vi "FGV Modbus Kommunikation OO.vi"(5 "Aktionen":T1=enum."lesen", 6 "error in":errorcluster caption="error out", 8 "IP-Adresse":string, 9 "Steuerung PNS (Eingang)":refnum<class "Steuerung PNS.lvclass">) -> (0 "Fehler (Ausgang)":errorcluster, 1 "Index":u8, 2 "Case Nr.":u8, 3 "Steuerung PNS (Ausgang)":refnum<class "Steuerung PNS.lvclass">, 4 "maxLoop":u8=10)   [LabVIEW 2020, in "PNS.lvlib" / "Komm Modbus.lvlib"]
uses:
  Komm Modbus.lvlib
  Aktionen FGV Komm MB.ctl
  ObjektKlassen/Steuerung PNS/Steuerung PNS.lvclass
  Aktionen FGV Grenzwerte.ctl
  Aktionen FGV Istwerte.ctl
  Aktion FGV AO PNS.ctl
  Aktion FGV Ventile manuell steuern.ctl
  Aktionen FGV Loopkennung.ctl
  PNS.lvlib
  Allgemein/allgemeine Sub-VIs.lvlib
  Modbus TypDef.lvlib
panel:
  out "x-y":u32
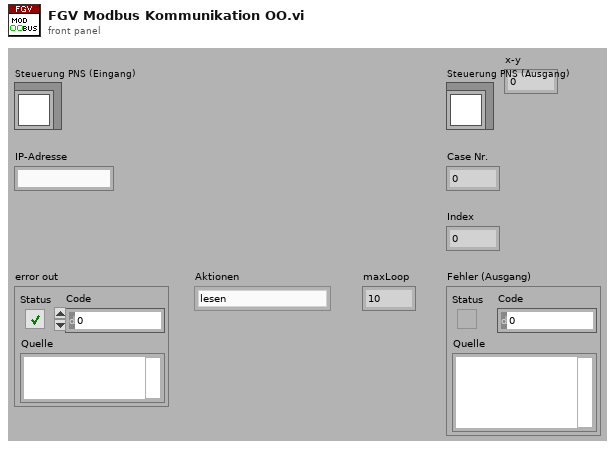
[diagram p1: front panel]
types:
  T1 = typedef "PNS.lvlib/Komm Modbus.lvlib/Modbus TypDef.lvlib/Aktionen FGV Komm MB.ctl" = enum16{"initialisieren", "lesen", "Verbindung herstellen", "Verbindung beenden", "Komm Modbus", "Sollwerte vorgeben", "change lang"}
  T2 = typedef "PNS.lvlib/Aktion FGV Ventile manuell steuern.ctl" = enum16{"lesen", "Ventile schalten"}
  T3 = typedef "PNS.lvlib/Aktion FGV AO PNS.ctl" = enum16{"lesen", "schreiben"}
  T4 = typedef "PNS.lvlib/Aktionen FGV Istwerte.ctl" = enum16{"lesen", "initialisieren", "schreiben", "Störungen"}
  T5 = typedef "PNS.lvlib/Aktionen FGV Grenzwerte.ctl" = enum16{"lesen", "Grenzw. schreiben", "Anweisungscode", "IP-Adresse", "laden", "speichern", "Anweisungscode vorgeben"}
  T6 = typedef "PNS.lvlib/Aktionen FGV Loopkennung.ctl" = enum16{"lesen", "schreiben"}
  T7 = typedef "Steuerung PNS.lvclass/Alarme.ctl" = cluster{"Alarm Filter max":u16, "Alarm Filter min":u16, "Alarm Ventilplatte max":u16, "Alarm Ventilplatte min":u16, "Alarm HL1 max":u16, "Alarm HL1 min":u16, "Alarm HL2 max":u16, "Alarm HL2 min":u16, "Alarm HL3 max":u16, "Alarm HL3 min":u16, "Alarm HL4 max":u16, "Alarm HL4 min":u16, "Alarm HL5 max":u16, "Alarm HL5 min":u16, "Alarm HL6 max":u16, "Alarm HL6 min":u16}
  T8 = typedef "Steuerung PNS.lvclass/Regler.ctl" = cluster{"Istwert":i16, "Sollwert":i16, "Alarm MIN":i16, "Alarm MAX":i16, "Regler sperren":i16, "Analog Ausgang":i16}[]
  T9 = typedef "Steuerung PNS.lvclass/Anlegengrenzwerte PNS.ctl" = cluster{"Filter:":T10, "Ventilplatte:":T10, "Heizleitung 1:":T10, "Heizleitung 2:":T10, "Heizleitung 3:":T10, "Heizleitung 4:":T10, "Heizleitung 5:":T10, "Heizleitung 6:":T10}
  T10 = typedef "Steuerung PNS.lvclass/Anlagengrenzwerte Parameteranzeige.ctl" = cluster{"Sollwert":T11, "Warn-Min":T11, "Warn-Max":T11, "Abschalt-Min":T11, "Abschalt-Max":T11, "Regler":u16, "AnlagenParameter":string}
  T11 = typedef "Zahlen-Eingabefeld.ctl" = sgl
  T12 = typedef "PNS.lvlib/PNS Geraetekennung.ctl" = cluster{"Loops":string[], "Gerätetype":string, "Loopkennung":u16[], "Seriennummer":string, "Geraetekennung":u16, "SoftWare Version":string, "LP Kennung":u16}
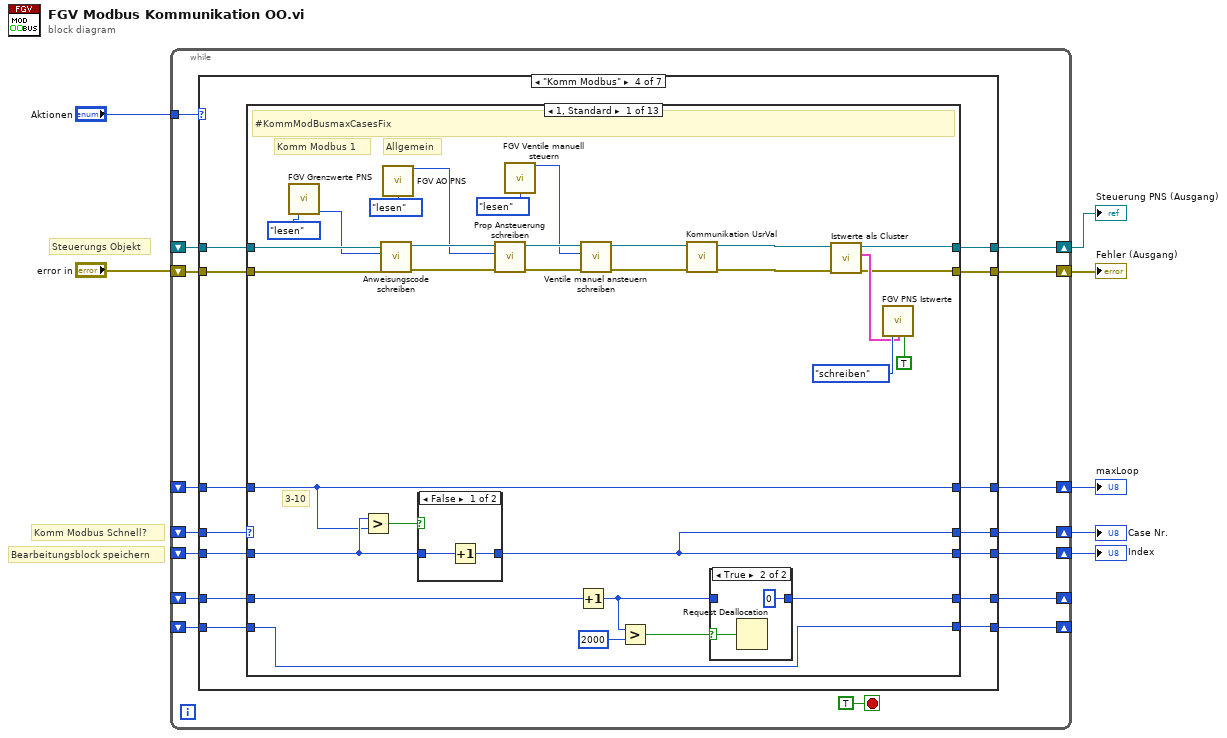
[diagram p0: block diagram]
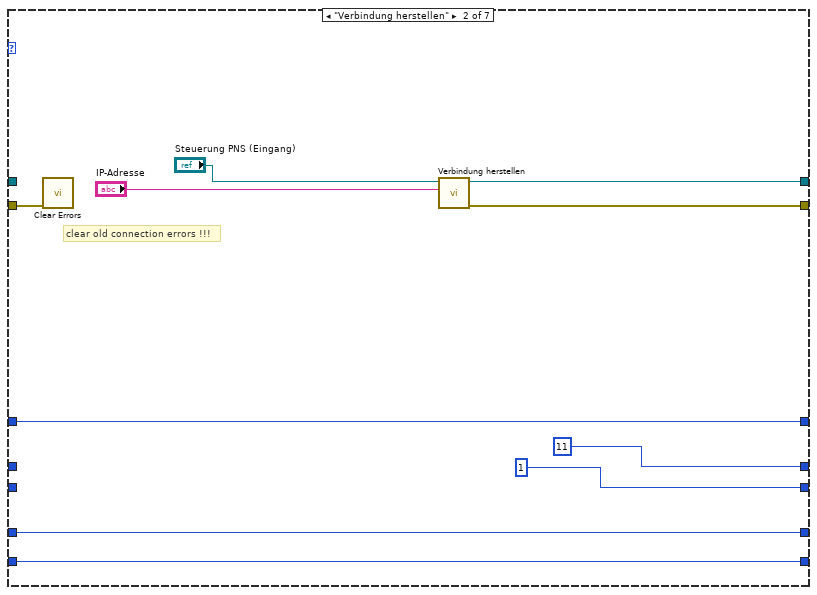
[diagram p3: hidden frame]
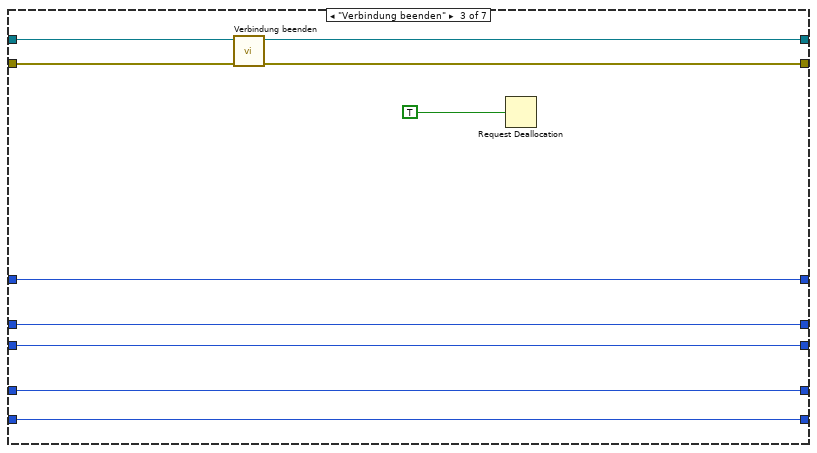
[diagram p4: hidden frame]
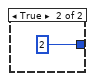
[diagram p6: hidden frame]
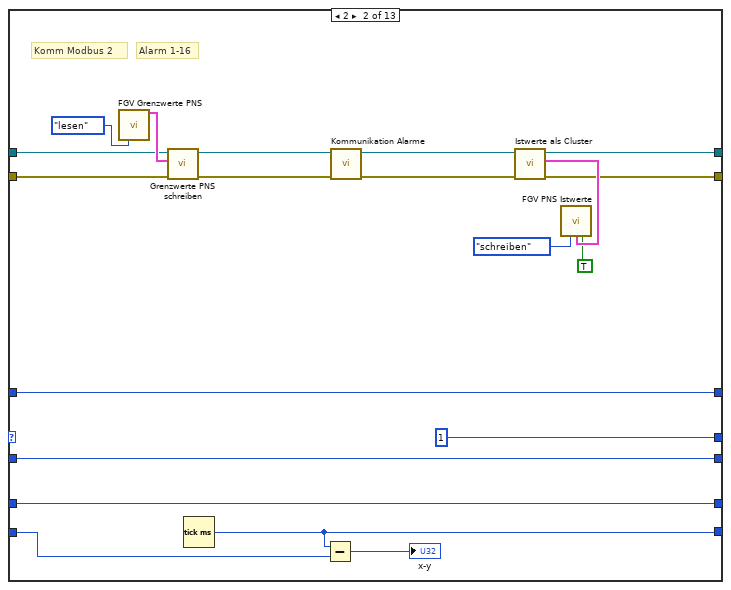
[diagram p7: hidden frame]
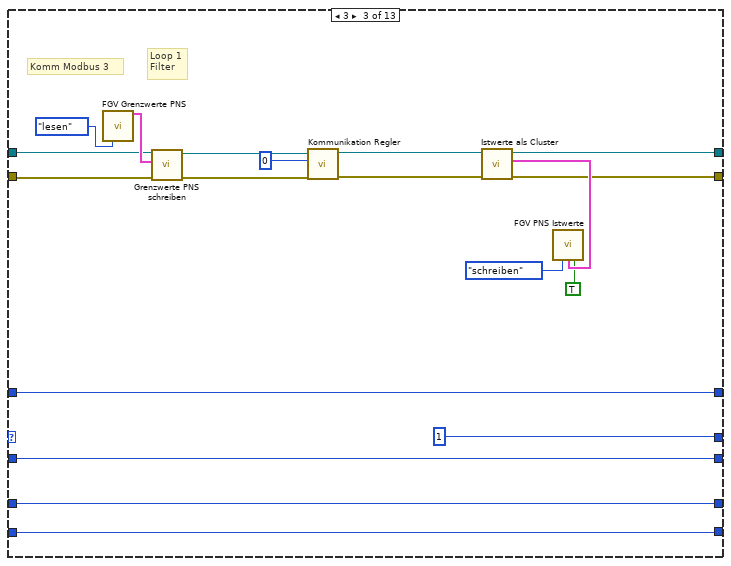
[diagram p8: hidden frame]
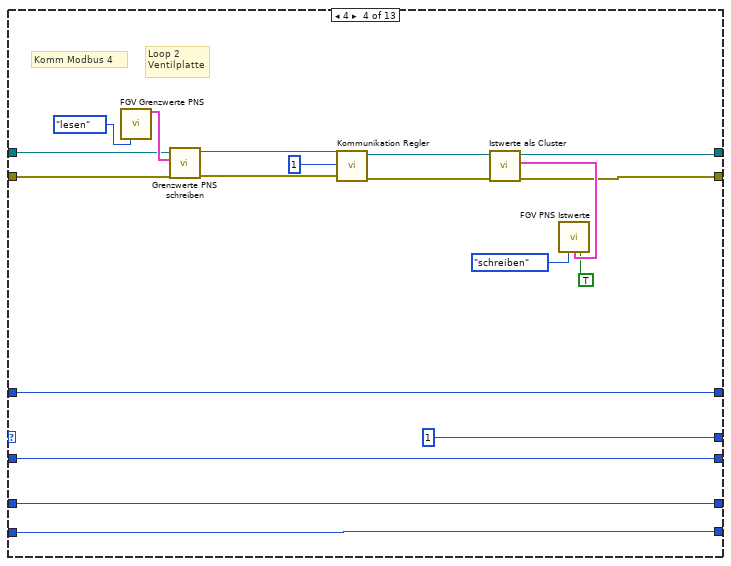
[diagram p9: hidden frame]
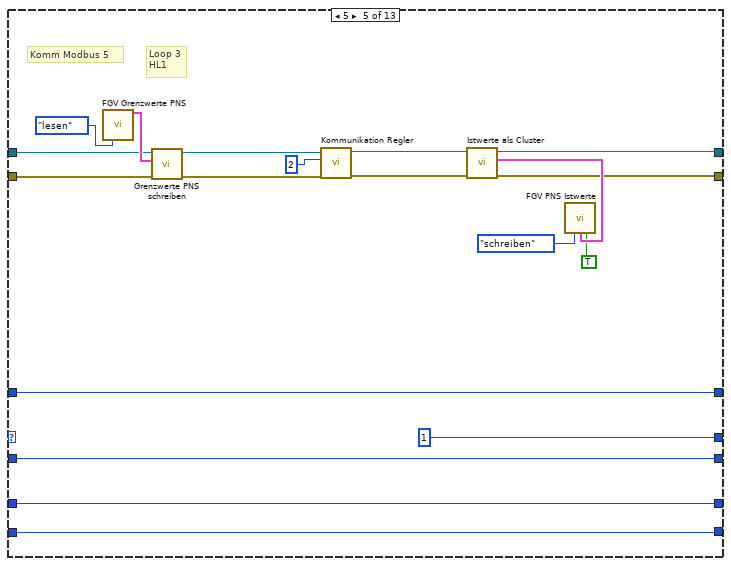
[diagram p10: hidden frame]
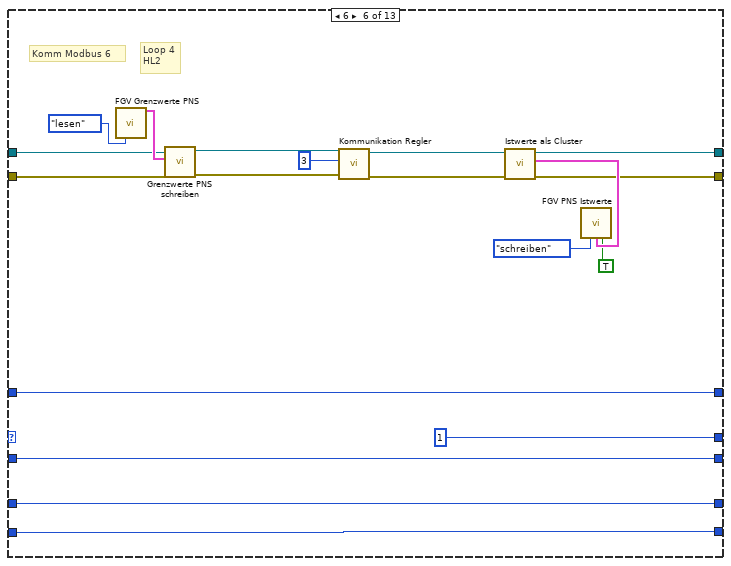
[diagram p11: hidden frame]
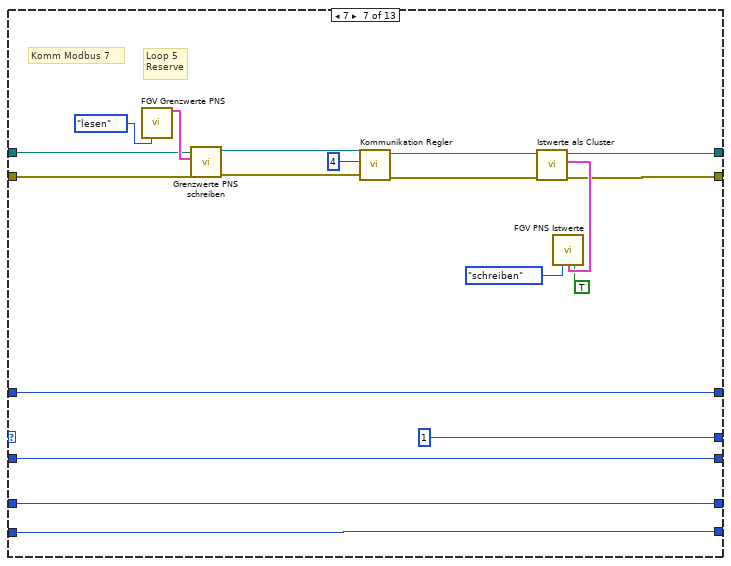
[diagram p12: hidden frame]
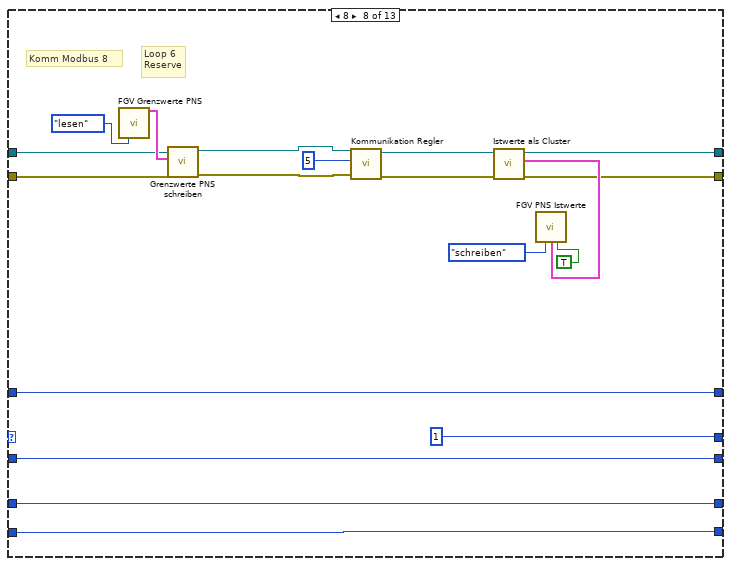
[diagram p13: hidden frame]
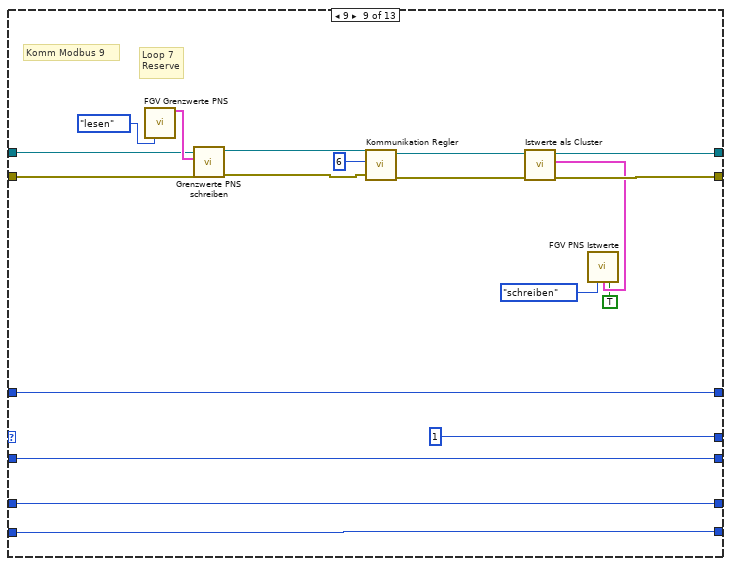
[diagram p14: hidden frame]
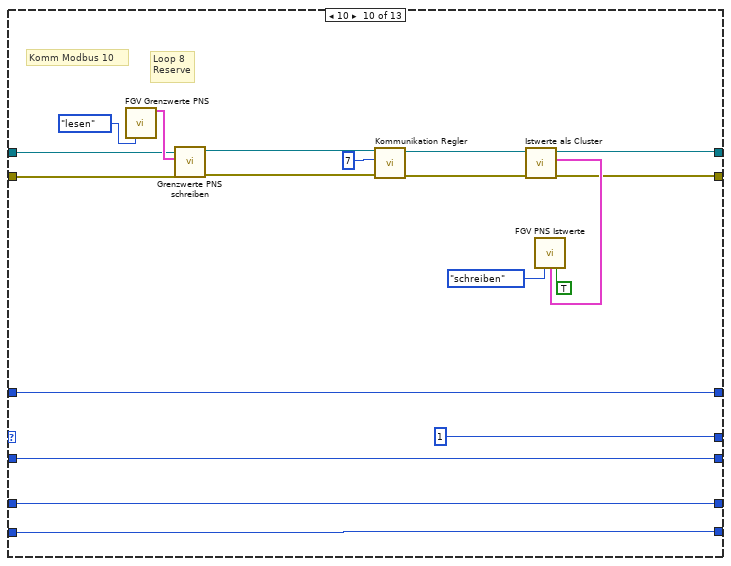
[diagram p15: hidden frame]
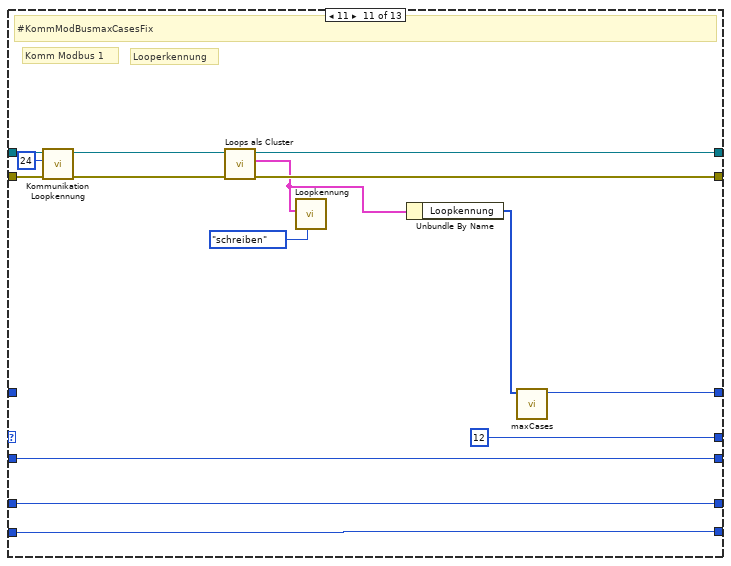
[diagram p16: hidden frame]
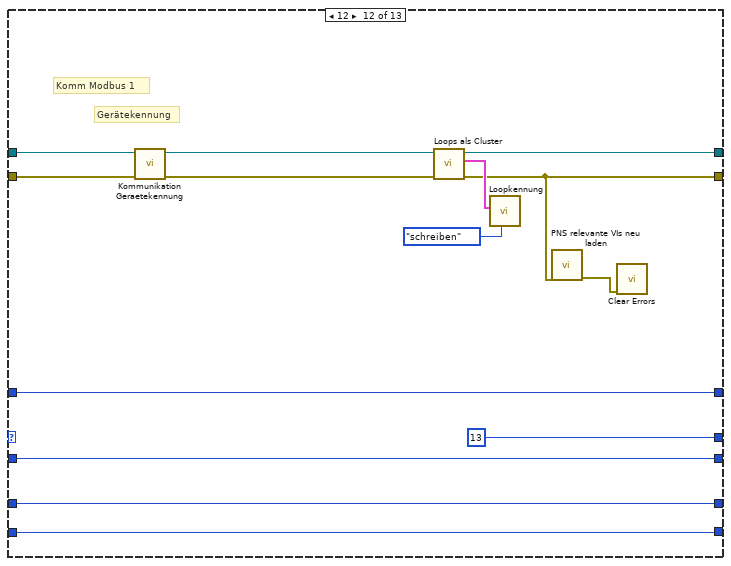
[diagram p17: hidden frame]
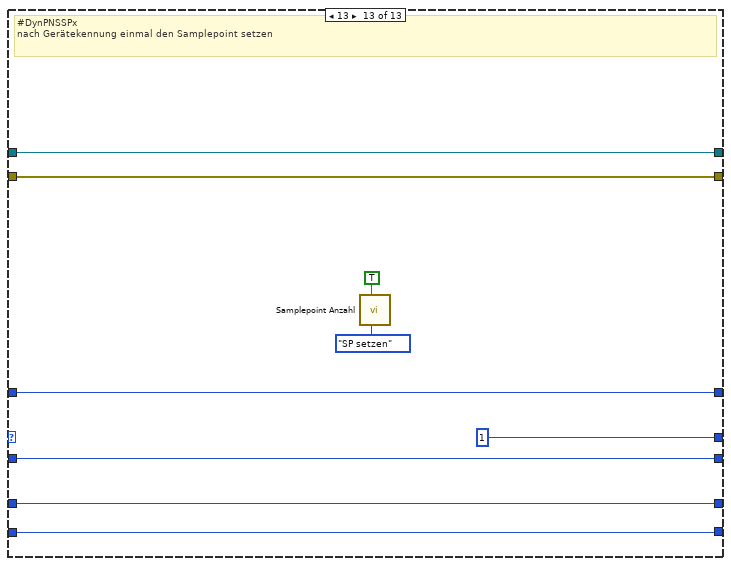
[diagram p18: hidden frame]
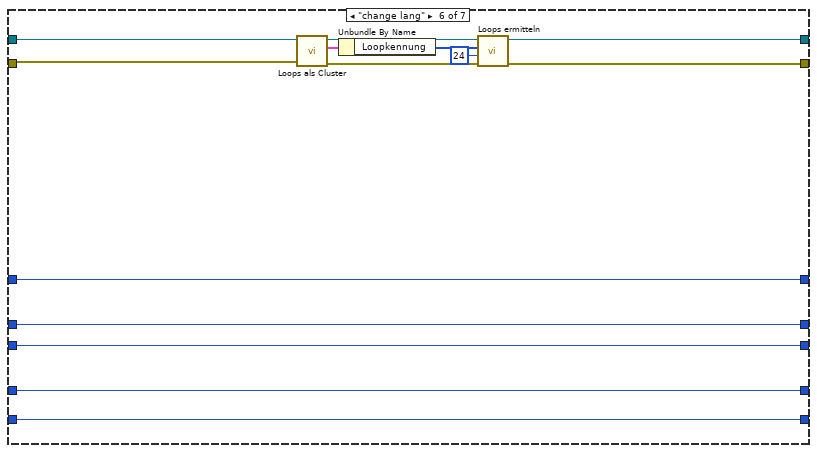
[diagram p20: hidden frame]
diagram:
  # "Bearbeitungsblock speichern"
  # "Komm Modbus Schnell?"
  # "Steuerungs Objekt"
  n1 = while {
    tunnel: "Aktionen" -> [w22]
    shift-right: [w21] -> w3
    shift-left: _ -> [w19]
    shift-right: [w20] -> w6
    shift-left: "error in" -> [w18]
    shift-right: [w16] -> w5
    shift-left: _ -> [w17]
    shift-right: [w15] -> w4
    shift-left: _ -> [w14]
    shift-right: [w13] -> _
    shift-left: _ -> [w12]
    shift-right: [w11] -> _
    shift-left: _ -> [w10]
    shift-right: [w9] -> w2
    shift-left: _ -> [w8]
    stop <- TRUE stop-if-true
    n2 = case shown="\"Komm Modbus\"" w22 {
      tunnel: [w30 w35 w45 w53 w318 w323 w338] -> w21
      tunnel: [w29 w36 w43 w64 w317 w321 w337] -> w20
      tunnel: w19 -> [w30 _ w42 w63 w318 w324 w338]
      tunnel: w18 -> [w29 w32 w44 w54 w317 w322 w337]
      tunnel: w17 -> [w28 _ w50 w59 w316 w331 w336]
      tunnel: [w28 u8 11 ("x") w50 w61 w316 w331 w336] -> w16
      tunnel: w14 -> [w27 _ w49 w62 w315 w330 w335]
      tunnel: [w27 u8 1 ("x") w49 w60 w315 w330 w335] -> w15
      tunnel: [w26 w39 w47 w57 w314 w332 w339] -> w13
      tunnel: w12 -> [w26 w39 w47 w58 w314 w332 w339]
      tunnel: [w25 w37 w46 w56 w313 w329 w334] -> w11
      tunnel: w10 -> [w25 w37 w46 w55 w313 w329 w334]
      tunnel: [w24 w31 w41 w52 w312 w319 w333] -> w9
      tunnel: w8 -> [w24 w31 w41 w51 w312 w319 w333]
      frame "lesen", Default {
      }
      frame "Verbindung herstellen" {
        # "clear old connection errors !!!"
        n3 = call <vilib>:"Clear Errors.vi"("error in (no error)"=w32) -> ()  [unwired: 5 in, 2 out]
        n4 = call "Verbindung herstellen.vi"("IP Adresse"="IP-Adresse", "Steuerung PNS (Eingang)"="Steuerung PNS (Eingang)") -> ("error out"=w36:errorcluster, "Steuerung PNS (Ausgang)"=w35:refnum<class "Steuerung PNS.lvclass">)  [unwired: 8 in]
      }
      frame "Verbindung beenden" {
        n5 = call "Verbindung beenden.vi"("error in (no error)"=w44, "Steuerung PNS Eingang"=w42) -> ("error out"=w43:errorcluster, "Steuerung PNS Ausgang"=w45:refnum<class "Steuerung PNS.lvclass">)  [unwired: 8 in]
        n6 = Request Deallocation(TRUE ("Flag")) -> ()
      }
      frame "Komm Modbus" {
        n7 = case shown="1, Standard" w59 {
          tunnel: [w78 w104 w124 w143 w162 w181 w200 w219 w240 w257 w278 w291 w306] -> w64
          tunnel: w63 -> [w85 w112 w132 w151 w170 w189 w208 w227 w246 w265 w284 w298 w307]
          tunnel: w62 -> [w93 w119 w138 w157 w176 w195 w214 w233 w252 w271 w287 w301 w310]
          tunnel: [w95 u8 1 ("x") u8 1 ("x") u8 1 ("x") u8 1 ("x") u8 1 ("x") u8 1 ("x") u8 1 ("x") u8 1 ("x") u8 1 ("x") u8 12 ("x") u8 13 ("x") u8 1 ("x")] -> w61
          tunnel: [w95 w119 w138 w157 w176 w195 w214 w233 w252 w271 w287 w301 w310] -> w60
          tunnel: w58 -> [w92 w120 w140 w159 w178 w197 w216 w235 w254 w273 w288 w302 w311]
          tunnel: [w89 w120 w140 w159 w178 w197 w216 w235 w254 w273 w288 w302 w311] -> w57
          tunnel: [w87 w118 w137 w156 w175 w194 w213 w232 w251 w270 w285 w299 w308] -> w56
          tunnel: w55 -> [w87 w116 w137 w156 w175 w194 w213 w232 w251 w270 w285 w299 w308]
          tunnel: w54 -> [w84 w109 w129 w149 w169 w188 w207 w226 w245 w264 w283 w297 w306]
          tunnel: [w82 w108 w128 w147 w166 w185 w204 w223 w242 w261 w280 w295 w307] -> w53
          tunnel: [w75 w102 w122 w141 w160 w179 w198 w217 w236 w255 w274 w289 w303] -> w52
          tunnel: w51 -> [w75 w102 w122 w141 w160 w179 w198 w217 w236 w255 _ w289 w303]
          frame 1, Default {
            # "3-10"
            # "Allgemein"
            # "Komm Modbus 1"
            # "#KommModBusmaxCasesFix"
            n8 = call "FGV Grenzwerte PNS.vi"("Aktionen FGV Grenzwerte"=Aktionen_FGV_Grenzwerte."lesen") -> ("Anweisungscode"=w76:u16)  [unwired: 12 in, 2 out]
            n9 = Greater?(x=w93, y=w75) -> (0:w94:bool)
            n10 = call-dynamic "Anweisungscode schreiben.vi"("error in (no error)"=w84, "Anweisungscode"=w76, "Steuerung PNS (Eingang)"=w85) -> ("error out"=w73:errorcluster, "Steuerung PNS (Ausgang)"=w74:refnum<class "Steuerung PNS.lvclass">)  [unwired: 7 in]
            n11 = call "FGV AO PNS.vi"("Aktion"=Aktion_FGV_AO_PNS."lesen") -> ("AO PROP"=w71:u16)  [unwired: 13 in, 1 out]
            n12 = case shown="False" w94 {
              tunnel: w93 -> [w100 _]
              tunnel: [w99 u8 2 ("Index")] -> w95
              frame False {
                n13 = Increment(x=w100) -> (x+1=w99:u8)
              }
              frame True {
              }
            }
            n14 = call-dynamic "Prop Ansteuerung schreiben.vi"("error in (no error)"=w73, "Propansteuerung"=w71, "Steuerung PNS (Eingang)"=w74) -> ("error out"=w68:errorcluster, "Steuerung PNS (Ausgang)"=w70:refnum<class "Steuerung PNS.lvclass">)  [unwired: 7 in]
            n15 = call "FGV Ventile manuell steuern.vi"("Aktion"=Aktion_FGV_Ventile_manuell_steuern."lesen") -> ("Ventile schalten"=w65:u32)  [unwired: 13 in, 1 out]
            n16 = Increment(x=w92) -> (x+1=w90:i32)
            n17 = call-dynamic "Ventile manuel ansteuern schreiben.vi"("error in (no error)"=w68, "Ventile steuern"=w65, "Steuerung PNS (Eingang)"=w70) -> ("error out"=w67:errorcluster, "Steuerung PNS (Ausgang)"=w69:refnum<class "Steuerung PNS.lvclass">)  [unwired: 7 in]
            n18 = Greater?(x=w90, y=2000) -> (0:w88:bool)
            n19 = call "Kommunikation UsrVal.vi"("error in (no error)"=w67, "Steuerung PNS Eingang"=w69) -> ("error out"=w79:errorcluster, "Steuerung PNS Ausgang"=w86:refnum<class "Steuerung PNS.lvclass">)  [unwired: 7 in, 1 out]
            n20 = case shown="True" w88 {
              selector: w88 -> [_ w97]
              tunnel: w90 -> [w96 _]
              tunnel: [w96 0] -> w89
              frame False {
              }
              frame True {
                n21 = Request Deallocation(w97) -> ()
              }
            }
            n22 = call "Istwerte als Cluster.vi"("error in (no error)"=w79, "Steuerung PNS Eingang"=w86) -> ("error out"=w78:errorcluster, "Cluster"=w80:cluster{"UsrVal":u16[], "Alarm":T7, "Regler":T8}, "Steuerung PNS Ausgang"=w82:refnum<class "Steuerung PNS.lvclass">)  [unwired: 7 in]
            n23 = call "FGV PNS Istwerte.vi"("Aktionen"=Aktionen_FGV_Istwerte."schreiben", "Cluster"=w80, "Speicher Freigabe"=TRUE) -> ()  [unwired: 9 in, 4 out]
          }
          frame 2 {
            # "Alarm 1-16"
            # "Komm Modbus 2"
            n24 = call "FGV Grenzwerte PNS.vi"("Aktionen FGV Grenzwerte"=Aktionen_FGV_Grenzwerte."lesen") -> ("Grenzwerte PNS 2"=w114:T9)  [unwired: 12 in, 2 out]
            n25 = call-dynamic "Grenzwerte PNS schreiben.vi"("error in (no error)"=w109, "Grenzwerte PNS"=w114, "Steuerung PNS (Eingang)"=w112) -> ("error out"=w110:errorcluster, "Steuerung PNS (Ausgang)"=w111:refnum<class "Steuerung PNS.lvclass">)  [unwired: 7 in]
            n26 = Tick Count (ms)() -> (millisecond timer value=w118:u32)
            n27 = Subtract(x=w118, y=w116) -> (x-y=→"x-y":u32)
            n28 = call "Kommunikation Alarme.vi"("error in (no error)"=w110, "Steuerung PNS Eingang"=w111) -> ("error out"=w105:errorcluster, "Steuerung PNS Ausgang"=w115:refnum<class "Steuerung PNS.lvclass">)  [unwired: 7 in, 1 out]
            n29 = call "Istwerte als Cluster.vi"("error in (no error)"=w105, "Steuerung PNS Eingang"=w115) -> ("error out"=w104:errorcluster, "Cluster"=w106:cluster{"UsrVal":u16[], "Alarm":T7, "Regler":T8}, "Steuerung PNS Ausgang"=w108:refnum<class "Steuerung PNS.lvclass">)  [unwired: 7 in]
            n30 = call "FGV PNS Istwerte.vi"("Aktionen"=Aktionen_FGV_Istwerte."schreiben", "Cluster"=w106, "Speicher Freigabe"=TRUE) -> ()  [unwired: 9 in, 4 out]
          }
          frame 3 {
            # "Loop 1\nFilter"
            # "Komm Modbus 3"
            n31 = call "FGV Grenzwerte PNS.vi"("Aktionen FGV Grenzwerte"=Aktionen_FGV_Grenzwerte."lesen") -> ("Grenzwerte PNS 2"=w133:T9)  [unwired: 12 in, 2 out]
            n32 = call-dynamic "Grenzwerte PNS schreiben.vi"("error in (no error)"=w129, "Grenzwerte PNS"=w133, "Steuerung PNS (Eingang)"=w132) -> ("error out"=w130:errorcluster, "Steuerung PNS (Ausgang)"=w131:refnum<class "Steuerung PNS.lvclass">)  [unwired: 7 in]
            n33 = call "Kommunikation Regler.vi"("error in (no error)"=w130, "Index"=u16 0, "Steuerung PNS Eingang"=w131) -> ("error out"=w125:errorcluster, "Steuerung PNS Ausgang"=w135:refnum<class "Steuerung PNS.lvclass">)  [unwired: 6 in, 1 out]
            n34 = call "Istwerte als Cluster.vi"("error in (no error)"=w125, "Steuerung PNS Eingang"=w135) -> ("error out"=w124:errorcluster, "Cluster"=w126:cluster{"UsrVal":u16[], "Alarm":T7, "Regler":T8}, "Steuerung PNS Ausgang"=w128:refnum<class "Steuerung PNS.lvclass">)  [unwired: 7 in]
            n35 = call "FGV PNS Istwerte.vi"("Aktionen"=Aktionen_FGV_Istwerte."schreiben", "Cluster"=w126, "Speicher Freigabe"=TRUE) -> ()  [unwired: 9 in, 4 out]
          }
          frame 4 {
            # "Loop 2\nVentilplatte"
            # "Komm Modbus 4"
            n36 = call "FGV Grenzwerte PNS.vi"("Aktionen FGV Grenzwerte"=Aktionen_FGV_Grenzwerte."lesen") -> ("Grenzwerte PNS 2"=w152:T9)  [unwired: 12 in, 2 out]
            n37 = call-dynamic "Grenzwerte PNS schreiben.vi"("error in (no error)"=w149, "Grenzwerte PNS"=w152, "Steuerung PNS (Eingang)"=w151) -> ("error out"=w148:errorcluster, "Steuerung PNS (Ausgang)"=w150:refnum<class "Steuerung PNS.lvclass">)  [unwired: 7 in]
            n38 = call "Kommunikation Regler.vi"("error in (no error)"=w148, "Index"=u16 1, "Steuerung PNS Eingang"=w150) -> ("error out"=w144:errorcluster, "Steuerung PNS Ausgang"=w154:refnum<class "Steuerung PNS.lvclass">)  [unwired: 6 in, 1 out]
            n39 = call "Istwerte als Cluster.vi"("error in (no error)"=w144, "Steuerung PNS Eingang"=w154) -> ("error out"=w143:errorcluster, "Cluster"=w145:cluster{"UsrVal":u16[], "Alarm":T7, "Regler":T8}, "Steuerung PNS Ausgang"=w147:refnum<class "Steuerung PNS.lvclass">)  [unwired: 7 in]
            n40 = call "FGV PNS Istwerte.vi"("Aktionen"=Aktionen_FGV_Istwerte."schreiben", "Cluster"=w145, "Speicher Freigabe"=TRUE) -> ()  [unwired: 9 in, 4 out]
          }
          frame 5 {
            # "Loop 3\nHL1"
            # "Komm Modbus 5"
            n41 = call "FGV Grenzwerte PNS.vi"("Aktionen FGV Grenzwerte"=Aktionen_FGV_Grenzwerte."lesen") -> ("Grenzwerte PNS 2"=w171:T9)  [unwired: 12 in, 2 out]
            n42 = call-dynamic "Grenzwerte PNS schreiben.vi"("error in (no error)"=w169, "Grenzwerte PNS"=w171, "Steuerung PNS (Eingang)"=w170) -> ("error out"=w167:errorcluster, "Steuerung PNS (Ausgang)"=w168:refnum<class "Steuerung PNS.lvclass">)  [unwired: 7 in]
            n43 = call "Kommunikation Regler.vi"("error in (no error)"=w167, "Index"=u16 2, "Steuerung PNS Eingang"=w168) -> ("error out"=w163:errorcluster, "Steuerung PNS Ausgang"=w173:refnum<class "Steuerung PNS.lvclass">)  [unwired: 6 in, 1 out]
            n44 = call "Istwerte als Cluster.vi"("error in (no error)"=w163, "Steuerung PNS Eingang"=w173) -> ("error out"=w162:errorcluster, "Cluster"=w164:cluster{"UsrVal":u16[], "Alarm":T7, "Regler":T8}, "Steuerung PNS Ausgang"=w166:refnum<class "Steuerung PNS.lvclass">)  [unwired: 7 in]
            n45 = call "FGV PNS Istwerte.vi"("Aktionen"=Aktionen_FGV_Istwerte."schreiben", "Cluster"=w164, "Speicher Freigabe"=TRUE) -> ()  [unwired: 9 in, 4 out]
          }
          frame 6 {
            # "Loop 4\nHL2"
            # "Komm Modbus 6"
            n46 = call "FGV Grenzwerte PNS.vi"("Aktionen FGV Grenzwerte"=Aktionen_FGV_Grenzwerte."lesen") -> ("Grenzwerte PNS 2"=w190:T9)  [unwired: 12 in, 2 out]
            n47 = call-dynamic "Grenzwerte PNS schreiben.vi"("error in (no error)"=w188, "Grenzwerte PNS"=w190, "Steuerung PNS (Eingang)"=w189) -> ("error out"=w186:errorcluster, "Steuerung PNS (Ausgang)"=w187:refnum<class "Steuerung PNS.lvclass">)  [unwired: 7 in]
            n48 = call "Kommunikation Regler.vi"("error in (no error)"=w186, "Index"=u16 3, "Steuerung PNS Eingang"=w187) -> ("error out"=w182:errorcluster, "Steuerung PNS Ausgang"=w192:refnum<class "Steuerung PNS.lvclass">)  [unwired: 6 in, 1 out]
            n49 = call "Istwerte als Cluster.vi"("error in (no error)"=w182, "Steuerung PNS Eingang"=w192) -> ("error out"=w181:errorcluster, "Cluster"=w183:cluster{"UsrVal":u16[], "Alarm":T7, "Regler":T8}, "Steuerung PNS Ausgang"=w185:refnum<class "Steuerung PNS.lvclass">)  [unwired: 7 in]
            n50 = call "FGV PNS Istwerte.vi"("Aktionen"=Aktionen_FGV_Istwerte."schreiben", "Cluster"=w183, "Speicher Freigabe"=TRUE) -> ()  [unwired: 9 in, 4 out]
          }
          frame 7 {
            # "Loop 5\nReserve"
            # "Komm Modbus 7"
            n51 = call "FGV Grenzwerte PNS.vi"("Aktionen FGV Grenzwerte"=Aktionen_FGV_Grenzwerte."lesen") -> ("Grenzwerte PNS 2"=w209:T9)  [unwired: 12 in, 2 out]
            n52 = call-dynamic "Grenzwerte PNS schreiben.vi"("error in (no error)"=w207, "Grenzwerte PNS"=w209, "Steuerung PNS (Eingang)"=w208) -> ("error out"=w205:errorcluster, "Steuerung PNS (Ausgang)"=w206:refnum<class "Steuerung PNS.lvclass">)  [unwired: 7 in]
            n53 = call "Kommunikation Regler.vi"("error in (no error)"=w205, "Index"=u16 4, "Steuerung PNS Eingang"=w206) -> ("error out"=w201:errorcluster, "Steuerung PNS Ausgang"=w211:refnum<class "Steuerung PNS.lvclass">)  [unwired: 6 in, 1 out]
            n54 = call "Istwerte als Cluster.vi"("error in (no error)"=w201, "Steuerung PNS Eingang"=w211) -> ("error out"=w200:errorcluster, "Cluster"=w202:cluster{"UsrVal":u16[], "Alarm":T7, "Regler":T8}, "Steuerung PNS Ausgang"=w204:refnum<class "Steuerung PNS.lvclass">)  [unwired: 7 in]
            n55 = call "FGV PNS Istwerte.vi"("Aktionen"=Aktionen_FGV_Istwerte."schreiben", "Cluster"=w202, "Speicher Freigabe"=TRUE) -> ()  [unwired: 9 in, 4 out]
          }
          frame 8 {
            # "Loop 6\nReserve"
            # "Komm Modbus 8"
            n56 = call "FGV Grenzwerte PNS.vi"("Aktionen FGV Grenzwerte"=Aktionen_FGV_Grenzwerte."lesen") -> ("Grenzwerte PNS 2"=w228:T9)  [unwired: 12 in, 2 out]
            n57 = call-dynamic "Grenzwerte PNS schreiben.vi"("error in (no error)"=w226, "Grenzwerte PNS"=w228, "Steuerung PNS (Eingang)"=w227) -> ("error out"=w224:errorcluster, "Steuerung PNS (Ausgang)"=w225:refnum<class "Steuerung PNS.lvclass">)  [unwired: 7 in]
            n58 = call "Kommunikation Regler.vi"("error in (no error)"=w224, "Index"=u16 5, "Steuerung PNS Eingang"=w225) -> ("error out"=w220:errorcluster, "Steuerung PNS Ausgang"=w230:refnum<class "Steuerung PNS.lvclass">)  [unwired: 6 in, 1 out]
            n59 = call "Istwerte als Cluster.vi"("error in (no error)"=w220, "Steuerung PNS Eingang"=w230) -> ("error out"=w219:errorcluster, "Cluster"=w221:cluster{"UsrVal":u16[], "Alarm":T7, "Regler":T8}, "Steuerung PNS Ausgang"=w223:refnum<class "Steuerung PNS.lvclass">)  [unwired: 7 in]
            n60 = call "FGV PNS Istwerte.vi"("Aktionen"=Aktionen_FGV_Istwerte."schreiben", "Cluster"=w221, "Speicher Freigabe"=TRUE) -> ()  [unwired: 9 in, 4 out]
          }
          frame 9 {
            # "Loop 7\nReserve"
            # "Komm Modbus 9"
            n61 = call "FGV Grenzwerte PNS.vi"("Aktionen FGV Grenzwerte"=Aktionen_FGV_Grenzwerte."lesen") -> ("Grenzwerte PNS 2"=w247:T9)  [unwired: 12 in, 2 out]
            n62 = call-dynamic "Grenzwerte PNS schreiben.vi"("error in (no error)"=w245, "Grenzwerte PNS"=w247, "Steuerung PNS (Eingang)"=w246) -> ("error out"=w243:errorcluster, "Steuerung PNS (Ausgang)"=w244:refnum<class "Steuerung PNS.lvclass">)  [unwired: 7 in]
            n63 = call "Kommunikation Regler.vi"("error in (no error)"=w243, "Index"=u16 6, "Steuerung PNS Eingang"=w244) -> ("error out"=w241:errorcluster, "Steuerung PNS Ausgang"=w249:refnum<class "Steuerung PNS.lvclass">)  [unwired: 6 in, 1 out]
            n64 = call "Istwerte als Cluster.vi"("error in (no error)"=w241, "Steuerung PNS Eingang"=w249) -> ("error out"=w240:errorcluster, "Cluster"=w238:cluster{"UsrVal":u16[], "Alarm":T7, "Regler":T8}, "Steuerung PNS Ausgang"=w242:refnum<class "Steuerung PNS.lvclass">)  [unwired: 7 in]
            n65 = call "FGV PNS Istwerte.vi"("Aktionen"=Aktionen_FGV_Istwerte."schreiben", "Cluster"=w238, "Speicher Freigabe"=TRUE) -> ()  [unwired: 9 in, 4 out]
          }
          frame 10 {
            # "Loop 8\nReserve"
            # "Komm Modbus 10"
            n66 = call "FGV Grenzwerte PNS.vi"("Aktionen FGV Grenzwerte"=Aktionen_FGV_Grenzwerte."lesen") -> ("Grenzwerte PNS 2"=w266:T9)  [unwired: 12 in, 2 out]
            n67 = call-dynamic "Grenzwerte PNS schreiben.vi"("error in (no error)"=w264, "Grenzwerte PNS"=w266, "Steuerung PNS (Eingang)"=w265) -> ("error out"=w262:errorcluster, "Steuerung PNS (Ausgang)"=w263:refnum<class "Steuerung PNS.lvclass">)  [unwired: 7 in]
            n68 = call "Kommunikation Regler.vi"("error in (no error)"=w262, "Index"=u16 7, "Steuerung PNS Eingang"=w263) -> ("error out"=w258:errorcluster, "Steuerung PNS Ausgang"=w268:refnum<class "Steuerung PNS.lvclass">)  [unwired: 6 in, 1 out]
            n69 = call "Istwerte als Cluster.vi"("error in (no error)"=w258, "Steuerung PNS Eingang"=w268) -> ("error out"=w257:errorcluster, "Cluster"=w259:cluster{"UsrVal":u16[], "Alarm":T7, "Regler":T8}, "Steuerung PNS Ausgang"=w261:refnum<class "Steuerung PNS.lvclass">)  [unwired: 7 in]
            n70 = call "FGV PNS Istwerte.vi"("Aktionen"=Aktionen_FGV_Istwerte."schreiben", "Cluster"=w259, "Speicher Freigabe"=TRUE) -> ()  [unwired: 9 in, 4 out]
          }
          frame 11 {
            # "Looperkennung"
            # "Komm Modbus 1"
            # "#KommModBusmaxCasesFix"
            n71 = call "Kommunikation Loopkennung.vi"("error in (no error)"=w283, "PNS SprachIndex (Seite)"=24, "Steuerung PNS Eingang"=w284) -> ("error out"=w279:errorcluster, "Steuerung PNS Ausgang"=w282:refnum<class "Steuerung PNS.lvclass">)  [unwired: 5 in, 2 out]
            n72 = call "Loops als Cluster.vi"("error in (no error)"=w279, "Steuerung PNS Eingang"=w282) -> ("error out"=w278:errorcluster, "LoopGeraetekennung"=w276:T12, "Steuerung PNS Ausgang"=w280:refnum<class "Steuerung PNS.lvclass">)  [unwired: 7 in]
            n73 = call "Loopkennung.vi"("Aktion"=Aktionen_FGV_Loopkennung."schreiben", "LoopGeraetekennung"=w276) -> ()  [unwired: 8 in, 2 out]
            n74 = Unbundle By Name(w276) -> ("Loopkennung"=w277:u16[])
            n75 = call "maxCases.vi"("Loopkennung"=w277) -> ("maxLoop"=w274:u8)  [unwired: 10 in]
          }
          frame 12 {
            # "Gerätekennung"
            # "Komm Modbus 1"
            n76 = call "Kommunikation Geraetekennung.vi"("error in (no error)"=w297, "Steuerung PNS Eingang"=w298) -> ("error out"=w293:errorcluster, "Steuerung PNS Ausgang"=w296:refnum<class "Steuerung PNS.lvclass">)  [unwired: 6 in, 2 out]
            n77 = call "Loops als Cluster.vi"("error in (no error)"=w293, "Steuerung PNS Eingang"=w296) -> ("error out"=w291:errorcluster, "LoopGeraetekennung"=w292:T12, "Steuerung PNS Ausgang"=w295:refnum<class "Steuerung PNS.lvclass">)  [unwired: 7 in]
            n78 = call "Loopkennung.vi"("Aktion"=Aktionen_FGV_Loopkennung."schreiben", "LoopGeraetekennung"=w292) -> ()  [unwired: 8 in, 2 out]
            n79 = call "PNS relevante VIs neu laden.vi"("Fehler (Eingang, kein Fehler)"=w291) -> ("Fehler (Ausgang)"=w290:errorcluster)  [unwired: 10 in]
            n80 = call <vilib>:"Clear Errors.vi"("error in (no error)"=w290) -> ()  [unwired: 5 in, 2 out]
          }
          frame 13 {
            # "#DynPNSSPx\nnach Gerätekennung einmal den Samplepoint setzen"
            n81 = call "Samplepoint Anzahl.vi"("Aktion"=enum16{"lesen", "Ref schreiben", "SP setzen"}."SP setzen", "PNS aktiv"=TRUE) -> ()  [unwired: 8 in, 2 out]
          }
        }
      }
      frame "Sollwerte vorgeben" {
      }
      frame "change lang" {
        n82 = call "Loops als Cluster.vi"("error in (no error)"=w322, "Steuerung PNS Eingang"=w324) -> ("error out"=w326:errorcluster, "LoopGeraetekennung"=w328:T12, "Steuerung PNS Ausgang"=w327:refnum<class "Steuerung PNS.lvclass">)  [unwired: 7 in]
        n83 = Unbundle By Name(w328) -> ("Loopkennung"=w325:u16[])
        n84 = call "Loops ermitteln.vi"("error in (no error)"=w326, "PNS SprachIndex (Seite)"=24, "Istwerte"=w325, "Steuerung PNS Eingang"=w327) -> ("error out"=w321:errorcluster, "Steuerung PNS Ausgang"=w323:refnum<class "Steuerung PNS.lvclass">)  [unwired: 4 in, 2 out]
      }
      frame "initialisieren" {
      }
    }
  }
  "Fehler (Ausgang)" <- w6
  "Case Nr." <- w5
  "Index" <- w4
  "Steuerung PNS (Ausgang)" <- w3
  "maxLoop" <- w2
